vi "Do.vi"(8 "error in (no error)":errorcluster, 10 "Actor in":refnum<class "Actor.lvclass">, 11 "Concrete Map Yaml Msg in":refnum<class "Concrete Map Yaml Msg.lvclass">) -> (0 "error out":errorcluster, 2 "Actor out":refnum<class "Actor.lvclass">)   [LabVIEW 2020, in "Yaml Model.lvlib" / "Concrete Map Yaml Msg.lvclass"]
doc: "(<B>Filename</B>: Actor Framework.lvlib:Message.lvclass:Do.vi)\n\nDefines what a message does when it is received by an actor. Generally, a message instructs an actor to invoke one of its methods.\n\nBy default, this method does nothing. A child class must override it to define behavior. Create a child class by using the Actor Framework Message Maker dialog box."
uses:
  Concrete Map Yaml Msg.lvclass
  E:/Project/Labview-Projects/Completed projects/Map Editor/Views/About View/About View Messages/Abstract Map Yaml Msg/Abstract Map Yaml Msg.lvclass
  <vilib>/ActorFramework/Actor/Actor.lvclass
  Yaml Model/Yaml Model.lvclass
  C:/Program Files/National Instruments/LabVIEW 2020/vi.lib/ActorFramework/Actor/Actor.lvclass
  Views/About View/About View Messages/Abstract Map Yaml Msg/Abstract Map Yaml Msg.lvclass
panel:
  # "NOTICE -- YOU MUST LEAVE THIS NOTICE IN PLACE.\n\nCopyright (c) 2017, LIANG LIU Shawn.Liu.cn@gmail.com\nAll rights reserved.\n\nRedistribution and use in source and binary forms, with or without modification, are permitted provided that the following conditions are met:\n-Redistributions of source code must retain the above copyright notice, this list of conditions and the following disclaimer.\n-Redistributions in binary form must reproduce the above copyright notice, this list of conditions and the following disclaimer in the documentation and/or other materials provided with the distribution.\n-Neither the name of the eLp nor the names of its contributors may be used to endorse or promote products derived from this software without specific prior written permission.\n\nTHIS SOFTWARE IS PROVIDED BY THE COPYRIGHT HOLDERS AND CONTRIBUTORS \"AS IS\" AND ANY EXPRESS OR IMPLIED WARRANTIES, INCLUDING, BUT NOT LIMITED TO, THE IMPLIED WARRANTIES OF MERCHANTABILITY AND FITNESS FOR A PARTICULAR PURPOSE ARE DISCLAIMED. IN NO EVENT SHALL THE COPYRIGHT HOLDER OR CONTRIBUTORS BE LIABLE FOR ANY DIRECT, INDIRECT, INCIDENTAL, SPECIAL, EXEMPLARY, OR CONSEQUENTIAL DAMAGES (INCLUDING, BUT NOT LIMITED TO, PROCUREMENT OF SUBSTITUTE GOODS OR SERVICES; LOSS OF USE, DATA, OR PROFITS; OR BUSINESS INTERRUPTION) HOWEVER CAUSED AND ON ANY THEORY OF LIABILITY, WHETHER IN CONTRACT, STRICT LIABILITY, OR TORT (INCLUDING NEGLIGENCE OR OTHERWISE) ARISING IN ANY WAY OUT OF THE USE OF THIS SOFTWARE, EVEN IF ADVISED OF THE POSSIBILITY OF SUCH DAMAGE."
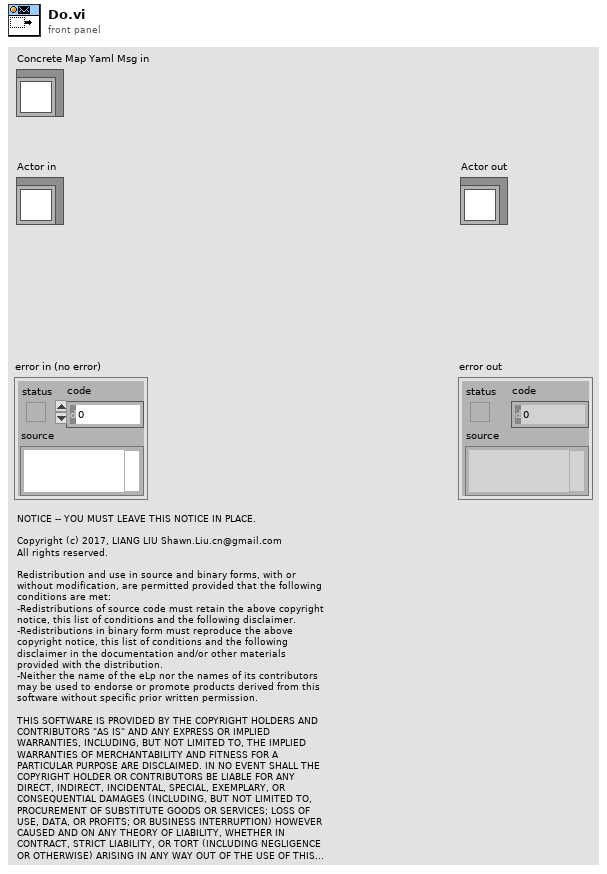
[diagram p1: front panel]
types:
  T1 = cluster{"Image":string, "Resolution":dbl, "Origin":cluster{"X":dbl, "Y":dbl, "R":dbl}, "Occupied Thresh":dbl, "Free Thresh":dbl, "Negate":bool}
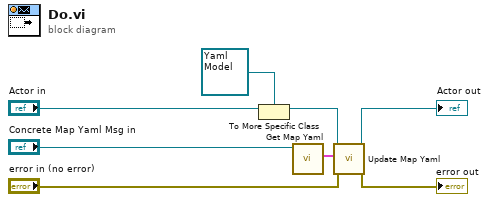
[diagram p0: block diagram]
diagram:
  n1 = To More Specific Class(target class=refnum<class "Yaml Model.lvclass"> refnum ("Yaml Model.lvlib:Yaml Model.lvclass"), reference="Actor in") -> (specific class reference=w5:refnum<class "Yaml Model.lvclass">)  [unwired: 1 in, 1 out]
  n2 = call "Get Map Yaml.vi"("Abstract Map Yaml Msg in"="Concrete Map Yaml Msg in") -> ("Map Yaml"=w3:T1)  [unwired: 9 in, 1 out]
  n3 = call "Update Map Yaml.vi"("error in (no error)"="error in (no error)", "Map Yaml"=w3, "Yaml Model in"=w5) -> ("error out"=→"error out":errorcluster, "Yaml Model out"=→"Actor out":refnum<class "Yaml Model.lvclass">)  [unwired: 7 in]
